vi "Set Center-Span - No Objects.vi"() -> ()   [LabVIEW 2012]
doc: "Sets the center and span (or start and stop) frequencies for a microwave sweep."
uses:
  Microwave.lvclass
  Math Operations/To Center and Span (frequency).vi
  Math Operations/To Start and Stop (frequency).vi
  Agilent PSG MXG Series/Agilent PSG MXG Series.lvlib
panel:
  in  "VISA resource name":refnum<visa-resource-name>
  out "Ready when\nblinking":bool
  out "Dwell":dbl[unit]=0.052000000000000005 caption="Steps"
  in  "Dwell Set":dbl[unit]=0.001
  out "Steps":i32=52
  out "Power":dbl=23.0
  in  "Steps Set":i32=101
  in  "Power Set":dbl=23.0
  out "Current Amplitude Mode":enum16{"Fixed", "Stepped Sweep", "List Sweep"}(ring)
  out "Current Frequency Mode":T1(ring)
  out "error out":errorcluster
  in  "Copy actual to set":bool
  in  "Populate fields with member data":bool
  out "Fake Microwave out":refnum<class "Microwave.lvclass">
  in  "error in (no error)":errorcluster
  in  "Fake Microwave in":refnum<class "Microwave.lvclass">
  out "Stop":dbl[unit] caption="Center"
  in  "Stop Set":dbl[unit]
  out "Start":dbl[unit] caption="Center"
  in  "Start Set":dbl[unit]
  in  "Read to Control":bool
  in  "Read":bool
  out "Span":dbl[unit]
  out "Center":dbl[unit]
  in  "Span Set":dbl[unit] caption="Span"
  in  "Center Set":dbl[unit] caption="Center"
  in  "Rf On/Off":bool caption="RF On/Off"
  in  "Exit":bool
  in  "Set":bool
  # "Set Center and Span\nfor Freq Sweep"
  # "For info purposes:"
  # "dBm"
  # "ms"
  # "GHz"
  # "GHz"
  # "GHz"
  # "GHz"
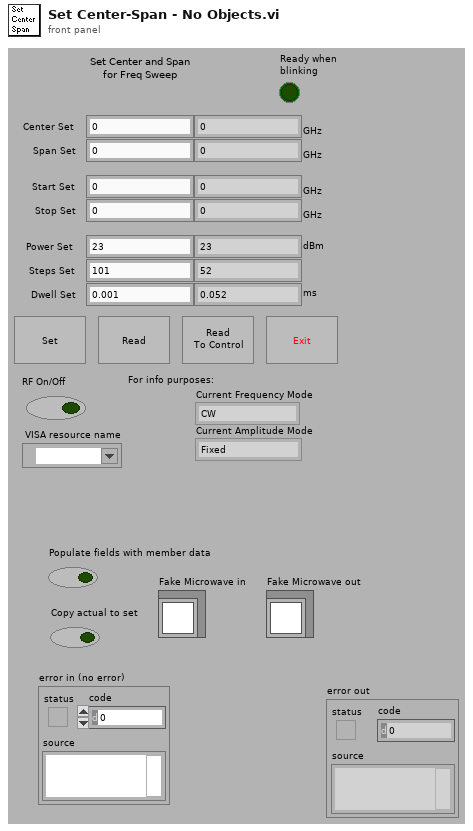
[diagram p1: front panel]
types:
  T1 = enum16{"CW", "Fixed", "Stepped Sweep", "List Sweep"}
  T2 = cluster{"Frequency Mode":u16, "Amplitude Mode":u16, "Frequency":dbl[unit], "Amplitude (dBm)":dbl, "Sweep Points":i32, "Sweep Dwell":dbl[unit], "Freq Sweep Start":dbl[unit], "Freq Sweep Stop":dbl[unit], "Amp Sweep Start (dBm)":dbl, "Amp Sweep Stop (dBm)":dbl, "rf on?":bool}
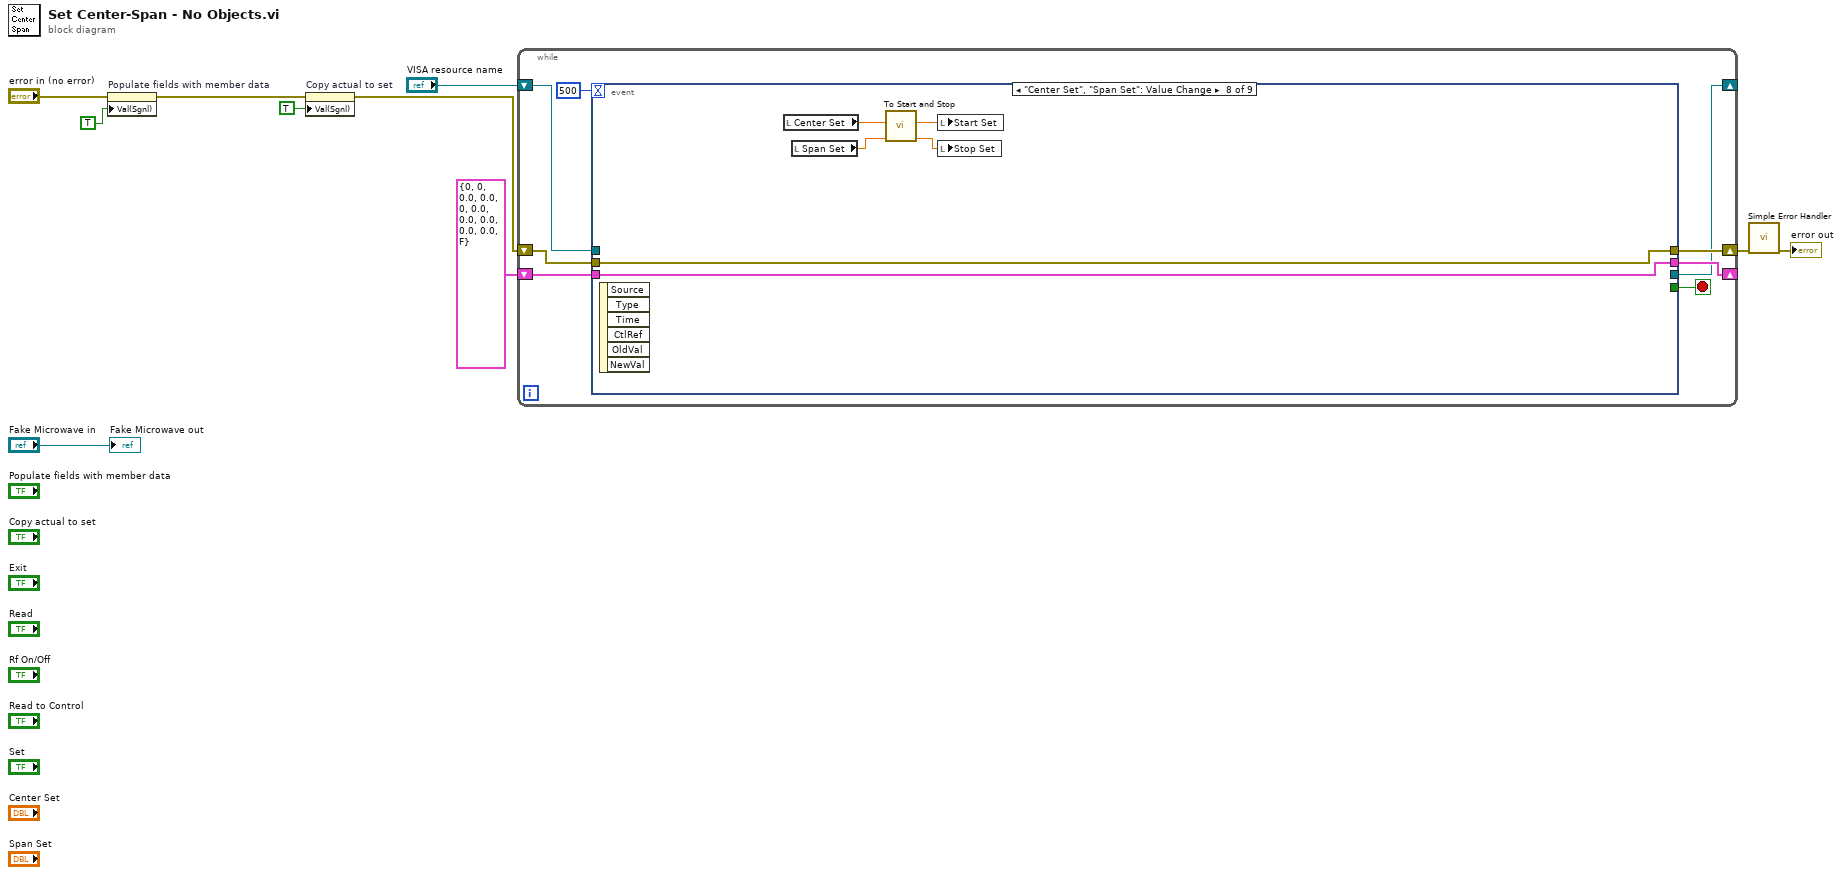
[diagram p0: block diagram]
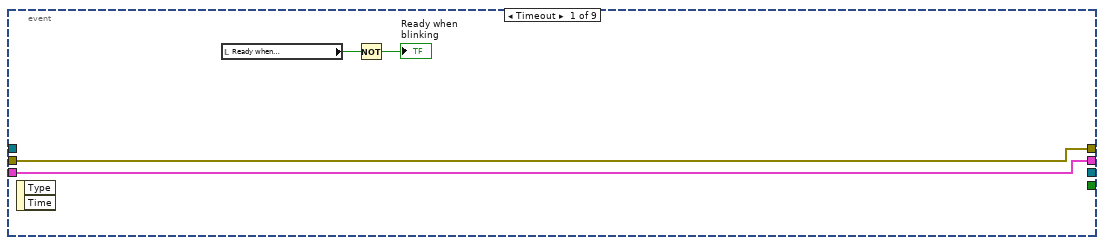
[diagram p2: hidden frame]
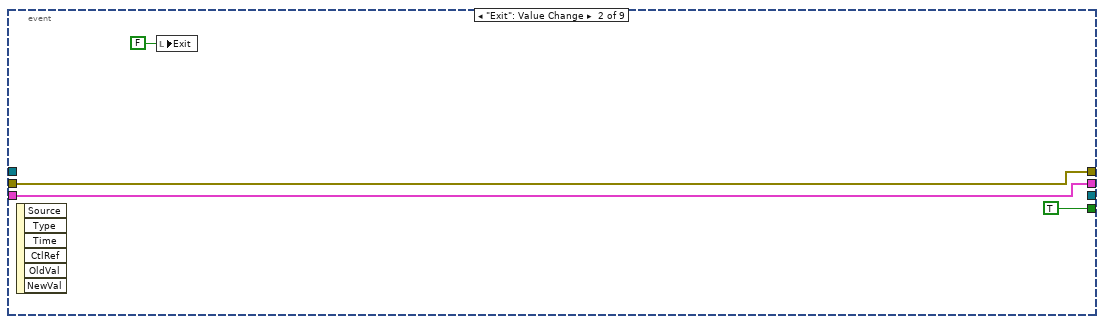
[diagram p3: hidden frame]
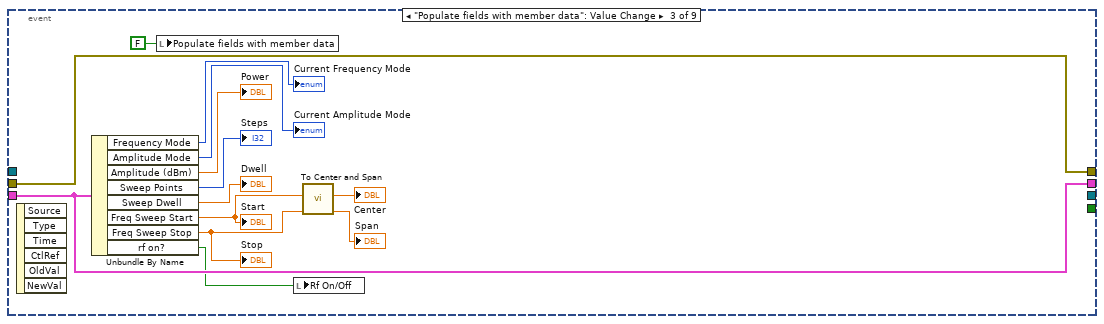
[diagram p4: hidden frame]
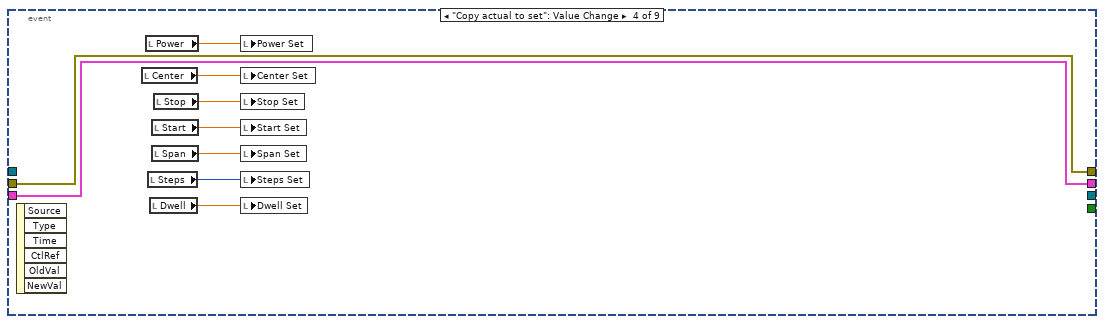
[diagram p5: hidden frame]
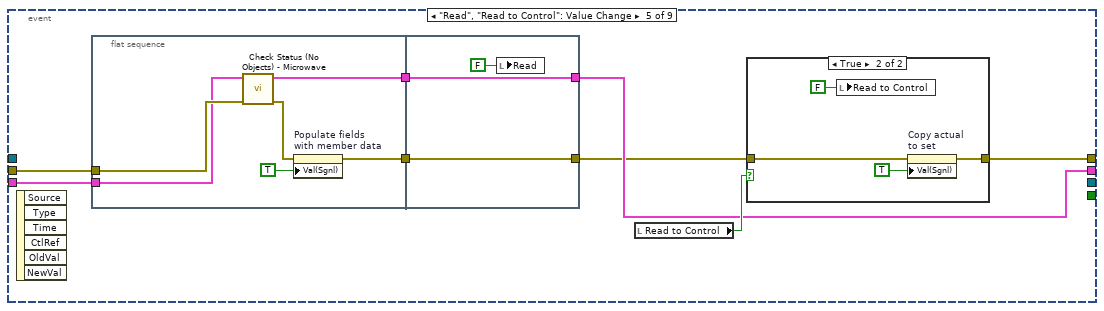
[diagram p6: hidden frame]
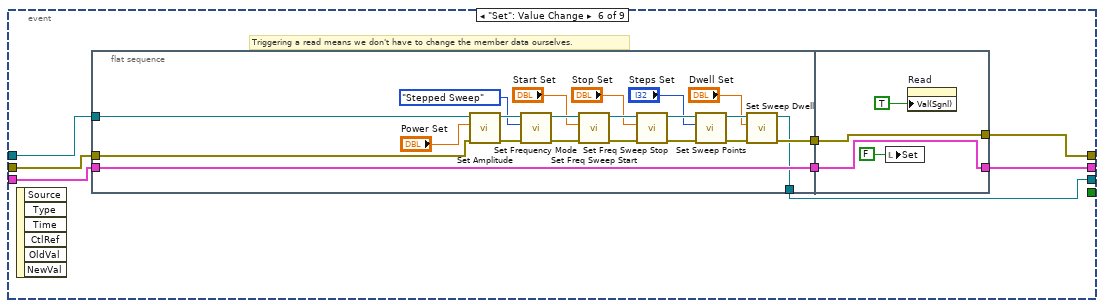
[diagram p8: hidden frame]
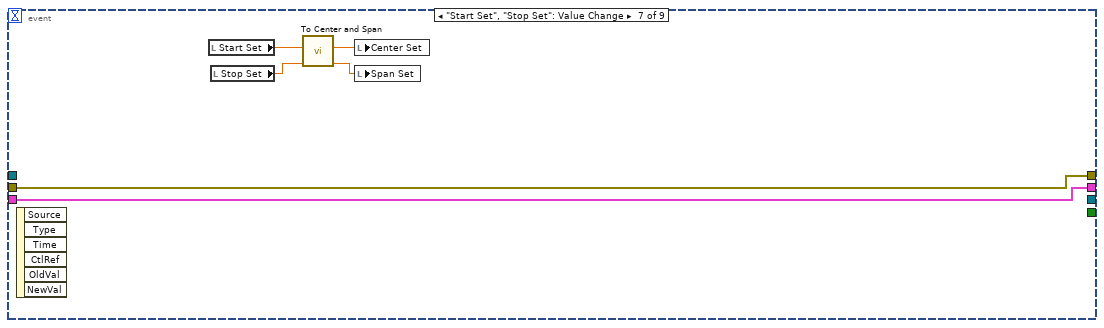
[diagram p9: hidden frame]
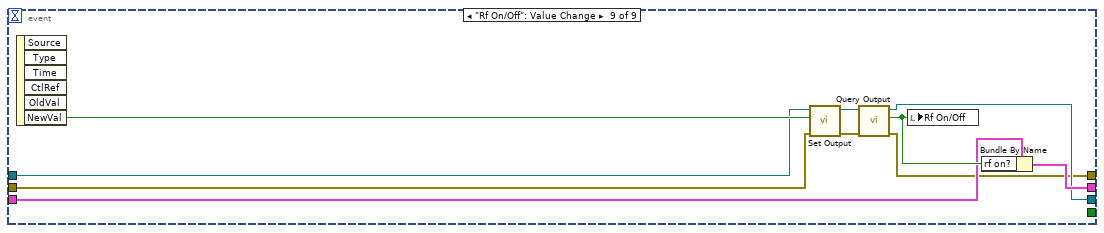
[diagram p10: hidden frame]
diagram:
  n1 = property on="Populate fields with member data" class="Bool (strict)"(error in="error in (no error)", "Val(Sgnl)"=TRUE ("Value (Signaling)")) -> (error out=w8:errorcluster)  [unwired: 1 in, 1 out]
  n2 = property on="Copy actual to set" class="Bool (strict)"(error in=w8, "Val(Sgnl)"=TRUE ("Value (Signaling)")) -> (error out=w5:errorcluster)  [unwired: 1 in, 1 out]
  n3 = while {
    shift-right: [w16] -> _
    shift-left: T2 {"Frequency Mode"=0, "Amplitude Mode"=0, "Frequency"=0.0, "Amplitude (dBm)"=0.0, "Sweep Points"=0, "Sweep Dwell"=0.0, "Freq Sweep Start"=0.0, "Freq Sweep Stop"=0.0, "Amp Sweep Start (dBm)"=0.0, "Amp Sweep Stop (dBm)"=0.0, "rf on?"=FALSE} ("Cluster of class private data") -> [w15]
    shift-right: [w17] -> w6
    shift-left: w5 -> [w14]
    shift-right: [w11] -> _
    shift-left: "VISA resource name" -> [w12]
    stop <- w18 stop-if-true
    n4 = event shown="[7] \"Center Set\", \"Span Set\": Value Change" {
      selector: _ -> [_ _ _ _ _ _ _ _ _]
      dyn-events: _ -> [_ _ _ _ _ _ _ _ _]
      timeout: 500 -> [_ _ _ _ _ _ _ _ _]
      tunnel: [_ TRUE _ _ _ _ _ _ _] -> w18
      tunnel: [w21 w23 w39 w47 w50 w76 w106 w110 w117] -> w17
      tunnel: w14 -> [w21 w23 w39 w47 w53 w77 w106 w110 w116]
      tunnel: [w22 w24 w38 w48 w54 w75 w107 w111 w123] -> w16
      tunnel: w15 -> [w22 w24 w38 w48 w55 w78 w107 w111 w119]
      tunnel: w12 -> [_ _ _ _ _ w74 _ _ w120]
      tunnel: [_ _ _ _ _ w71 _ _ w118] -> w11
      event Timeout {
        n5 = event-data() -> ()  [unwired: 3 out]
        n6 = local read "Ready when\nblinking"() -> (w19:bool)
        n7 = Not(x=w19) -> (.not. x?=→"Ready when\nblinking":bool)
      }
      event "Exit": Value Change {
        n8 = event-data() -> ()  [unwired: 7 out]
        n9 = local write "Exit"(FALSE ("Exit")) -> ()
      }
      event "Populate fields with member data": Value Change {
        n10 = event-data() -> ()  [unwired: 7 out]
        n11 = Unbundle By Name(w38) -> ("Frequency Mode"=→"Current Frequency Mode":u16, "Amplitude Mode"=→"Current Amplitude Mode":u16, "Amplitude (dBm)"=→"Power":dbl, "Sweep Points"=→"Steps":i32, "Sweep Dwell"=→"Dwell":dbl[unit], "Freq Sweep Start"=w32:dbl[unit], "Freq Sweep Stop"=w31:dbl[unit], "rf on?"=w28:bool)
        "Start" <- w32
        "Stop" <- w31
        n12 = local write "Populate fields with member data"(FALSE ("Populate fields with member data")) -> ()
        n13 = local write "Rf On/Off"(w28) -> ()
        n14 = call-poly "To Center and Span.vi"("stop"=w31, "start"=w32) -> ("span"=→"Span":dbl[unit], "center"=→"Center":dbl[unit])  [unwired: 4 out]
      }
      event "Copy actual to set": Value Change {
        n15 = event-data() -> ()  [unwired: 7 out]
        n16 = local read "Center"() -> (w46:dbl[unit])
        n17 = local read "Power"() -> (w42:dbl)
        n18 = local read "Steps"() -> (w41:i32)
        n19 = local read "Dwell"() -> (w40:dbl[unit])
        n20 = local read "Start"() -> (w44:dbl[unit])
        n21 = local read "Span"() -> (w45:dbl[unit])
        n22 = local read "Stop"() -> (w43:dbl[unit])
        n23 = local write "Power Set"(w42) -> ()
        n24 = local write "Center Set"(w46) -> ()
        n25 = local write "Stop Set"(w43) -> ()
        n26 = local write "Start Set"(w44) -> ()
        n27 = local write "Span Set"(w45) -> ()
        n28 = local write "Steps Set"(w41) -> ()
        n29 = local write "Dwell Set"(w40) -> ()
      }
      event "Read", "Read to Control": Value Change {
        n30 = event-data() -> ()  [unwired: 7 out]
        n31 = flat-sequence {
          tunnel: w55 -> [w57]
          tunnel: w53 -> [w61]
          tunnel: [w62] -> w52
          tunnel: [w58] -> w51
          tunnel: [w64] -> w49
          tunnel: [w65] -> w54
          tunnel: w52 -> [w65]
          tunnel: w51 -> [w64]
          frame #0 {
            n32 = call "Check Status (No Objects) - Microwave.vi"("error in (no error)"=w61, "Cluster In"=w57) -> ("error out"=w59:errorcluster, "Cluster Out"=w62:T2)  [unwired: 6 in, 2 out]
            n33 = property on="Populate fields \nwith member data" class="Bool (strict)"(error in=w59, "Val(Sgnl)"=TRUE ("Value (Signaling)")) -> (error out=w58:errorcluster)  [unwired: 1 in, 1 out]
          }
          frame #1 {
            n34 = local write "Read"(FALSE ("Read")) -> ()
          }
        }
        n35 = local read "Read to Control"() -> (w56:bool)
        n36 = case shown="True" w56 {
          tunnel: w49 -> [w66 w69]
          tunnel: [w66 w68] -> w50
          frame False {
          }
          frame True {
            n37 = local write "Read to Control"(FALSE ("Read to Control")) -> ()
            n38 = property on="Copy actual \nto set" class="Bool (strict)"(error in=w69, "Val(Sgnl)"=TRUE ("Value (Signaling)")) -> (error out=w68:errorcluster)  [unwired: 1 in, 1 out]
          }
        }
      }
      event "Set": Value Change {
        # "Triggering a read means we don't have to change the member data ourselves."
        n39 = event-data() -> ()  [unwired: 7 out]
        n40 = flat-sequence {
          tunnel: w78 -> [w82]
          tunnel: w77 -> [w80]
          tunnel: w74 -> [w83]
          tunnel: [w82] -> w73
          tunnel: [w81] -> w72
          tunnel: [w79] -> w71
          tunnel: [w102] -> w76
          tunnel: [w101] -> w75
          tunnel: w73 -> [w101]
          tunnel: w72 -> [w102]
          frame #0 {
            n41 = call "Set Amplitude.vi"("error in (no error)"=w80, "Amplitude (dBm)"="Power Set", "VISA resource name"=w83) -> ("error out"=w94:errorcluster, "VISA resource name out"=w99:refnum<visa-resource-name>)  [unwired: 7 out]
            n42 = call "Set Frequency Mode.vi"("error in (no error)"=w94, "Frequency Mode"=T1."Stepped Sweep", "VISA resource name"=w99) -> ("error out"=w93:errorcluster, "VISA resource name out"=w98:refnum<visa-resource-name>)  [unwired: 7 out]
            n43 = call "Set Freq Sweep Start.vi"("error in (no error)"=w93, "Frequency Sweep Start"="Start Set", "VISA resource name"=w98) -> ("error out"=w92:errorcluster, "VISA resource name out"=w97:refnum<visa-resource-name>)  [unwired: 7 out]
            n44 = call "Set Freq Sweep Stop.vi"("error in (no error)"=w92, "Frequency Sweep Stop"="Stop Set", "VISA resource name"=w97) -> ("error out"=w91:errorcluster, "VISA resource name out"=w96:refnum<visa-resource-name>)  [unwired: 7 out]
            n45 = call "Set Sweep Points.vi"("error in (no error)"=w91, "Number of Sweep Points"="Steps Set", "VISA resource name"=w96) -> ("error out"=w90:errorcluster, "VISA resource name out"=w95:refnum<visa-resource-name>)  [unwired: 7 out]
            n46 = call "Set Sweep Dwell.vi"("error in (no error)"=w90, "Sweep Dwell Time"="Dwell Set", "VISA resource name"=w95) -> ("error out"=w81:errorcluster, "VISA resource name out"=w79:refnum<visa-resource-name>)  [unwired: 7 out]
          }
          frame #1 {
            n47 = local write "Set"(FALSE ("Set")) -> ()
            n48 = property on="Read" class="Bool (strict)"("Val(Sgnl)"=TRUE ("Value (Signaling)")) -> ()  [unwired: 2 in, 2 out]
          }
        }
      }
      event "Start Set", "Stop Set": Value Change {
        n49 = event-data() -> ()  [unwired: 7 out]
        n50 = local read "Start Set"() -> (w105:dbl[unit])
        n51 = local read "Stop Set"() -> (w104:dbl[unit])
        n52 = call-poly "To Center and Span.vi"("stop"=w104, "start"=w105) -> ("span"=w108:dbl[unit], "center"=w109:dbl[unit])  [unwired: 4 out]
        n53 = local write "Center Set"(w109) -> ()
        n54 = local write "Span Set"(w108) -> ()
      }
      event "Center Set", "Span Set": Value Change {
        n55 = event-data() -> ()  [unwired: 7 out]
        n56 = local read "Center Set"() -> (w115:dbl[unit])
        n57 = local read "Span Set"() -> (w114:dbl[unit])
        n58 = call-poly "To Start and Stop.vi"("span"=w114, "center"=w115) -> ("stop"=w112:dbl[unit], "start"=w113:dbl[unit])  [unwired: 4 out]
        n59 = local write "Start Set"(w113) -> ()
        n60 = local write "Stop Set"(w112) -> ()
      }
      event "Rf On/Off": Value Change {
        n61 = event-data() -> ("NewVal"=w121:bool)  [unwired: 6 out]
        n62 = call "Set Output.vi"("error in (no error)"=w116, "Output On"=w121, "VISA resource name"=w120) -> ("error out"=w124:errorcluster, "VISA resource name out"=w125:refnum<visa-resource-name>)  [unwired: 7 out]
        n63 = call "Query Output.vi"("error in (no error)"=w124, "VISA resource name"=w125) -> ("error out"=w117:errorcluster, "Output On?"=w122:bool, "VISA resource name out"=w118:refnum<visa-resource-name>)  [unwired: 7 out]
        n64 = local write "Rf On/Off"(w122) -> ()
        n65 = Bundle By Name(cluster=w119, "rf on?"=w122) -> (w123:T2)
      }
    }
  }
  n66 = call <vilib>:"Simple Error Handler.vi"("error in (no error)"=w6) -> ("error out"=→"error out":errorcluster)  [unwired: 1 in, 7 out]
  "Fake Microwave out" <- "Fake Microwave in"
